vi "FL_Preprocess_and_save_incrementally.vi"(0 "Temporary file output path":path, 1 "Loop iteration":i32, 2 "Mouse face dir. swap":bool, 3 "Loop speed in ms":u16, 4 "Save every N seconds":u32=15, 5 "error in (no error)":errorcluster, 6 "Filter type":u16(ring)=5 items=["None", "Kalman 0.50", "Kalman 0.30", "Kalman 0.12", "Savitzky-Golay 3/5", "Savitzky-Golay 3/11", "Savitzky-Golay 3/31"], 7 "Sensor read input":T3(array[cluster]), 8 "Offset":sgl, 9 "tdms file in":refnum<k34>, 10 "Pixels per mm":dbl, 11 "Data flow controls in":T2, 12 "Diagram at recording bounds":T1, 13 "Sensor board size":string="Small") -> (14 "Eff. save interval":sgl, 15 "Latest sensor output (decoded)":string[][](array[string]), 16 "Fire TTL":bool, 17 "TTL out N":u8, 18 "Current TTL status":u8, 19 "error out":errorcluster)   [LabVIEW 2018, in "Tracker.lvlib"]
uses:
  Tracker.lvlib
  SW_Globals.vi
  <vilib>/Utility/miscctls.llb/LVBoundsTypeDef.ctl
  <vilib>/Utility/file.llb/Write Delimited Spreadsheet (string).vi
panel:
  out "Bytes return count":u32
  out "VISA error out":errorcluster
  out "Output to the external terminal":string
  in  "Max chunk size":i64=100000
  in  "Number of the file chunk":u32
  out "Chunk size (in bytes)":i64
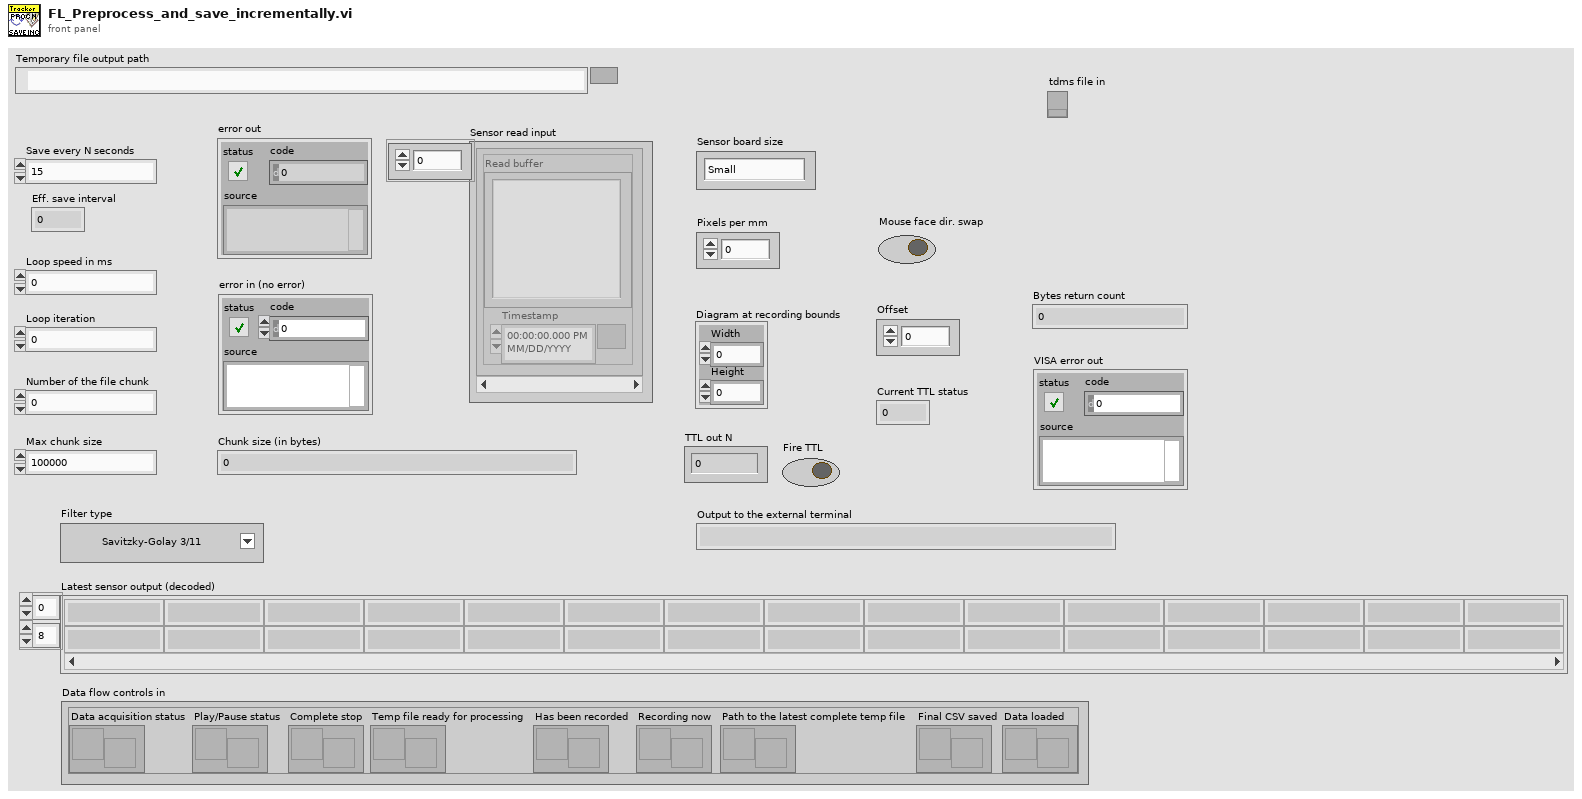
[diagram p1: front panel]
types:
  T1 = typedef "LVBoundsTypeDef.ctl" = cluster{"Width":u32, "Height":u32}
  T2 = cluster{"Data acquisition status":refnum<notifier>, "Play/Pause status":refnum<notifier>, "Complete stop":refnum<notifier>, "Temp file ready for processing":refnum<notifier>, "Has been recorded":refnum<notifier>, "Recording now":refnum<notifier>, "Path to the latest complete temp file":refnum<notifier>, "Final CSV saved":refnum<notifier>, "Data loaded":refnum<notifier>}
  T3 = cluster{"Read buffer":string, "Timestamp":timestamp}[]
  T4 = cluster{"ms since ON":u32, "delta time":u32, "X1":sgl, "Y1":sgl, "X2":sgl, "Y2":sgl, "TTL inputs":u8, "TTL outputs":u8, "Frame timestamp":timestamp, "Frame OK":bool}
  T5 = cluster{"X1 filtered":dbl, "Y1 filtered":dbl, "X2 filtered":dbl, "Y2 filtered":dbl, "X1 raw":dbl, "Y1 raw":dbl, "X2 raw":dbl, "Y2 raw":dbl}
  T6 = cluster{"R from center":dbl, "sin(a)":dbl, "Mouse Xc":dbl, "Mouse Yc":dbl, "X1-X2":dbl, "Y1-Y2":dbl, "Cage Xc":dbl, "Cage Yc":dbl}
  T7 = cluster{"R from center":dbl, "phi (mouse angular position in the cage)":dbl, "alpha (mouse rot. angle)":sgl, "X":dbl, "Y":dbl, "theta (from center towards mouse)":dbl, "beta (cage rot. against mouse)":sgl, "w (mouse angle to wall)":dbl}
  T8 = cluster{"Zone[1]":bool, "Zone[2]":bool, "Zone[3]":bool, "Zone[4]":bool, "Zone[5]":bool, "Zone[6]":bool, "Zone[7]":bool, "Zone[8]":bool, "Zone[9]":bool, "Zone[10]":bool, "Zone[11]":bool, "Zone[12]":bool, "Zone[13]":bool}
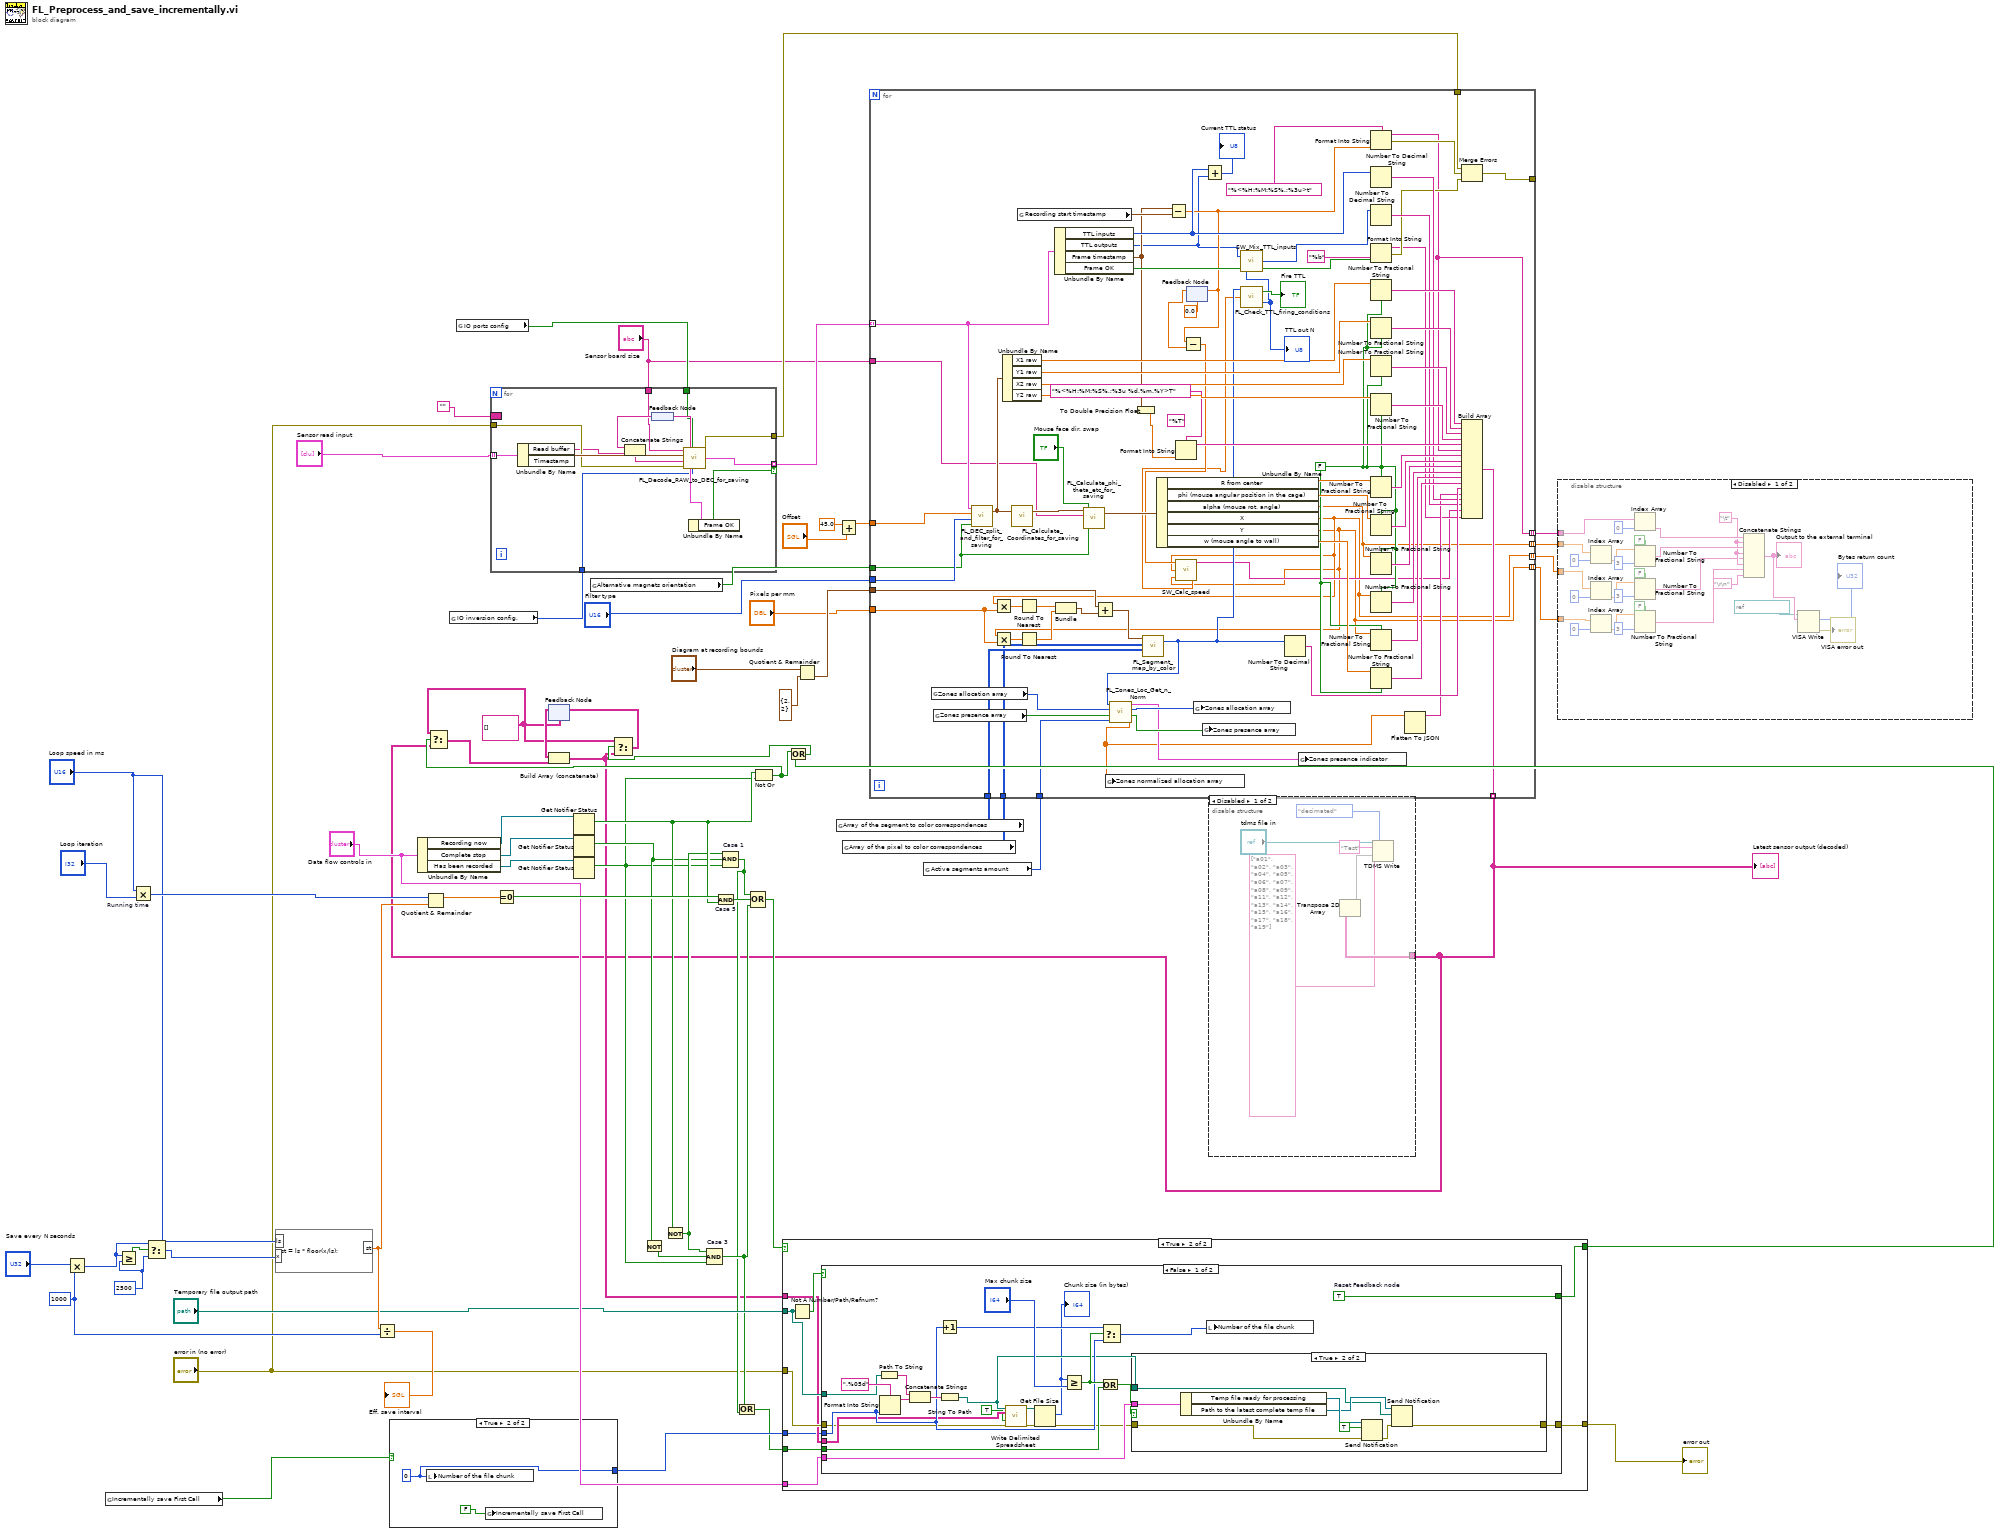
[diagram p0: block diagram]
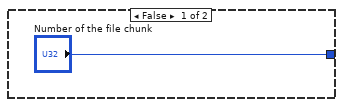
[diagram p4: hidden frame]
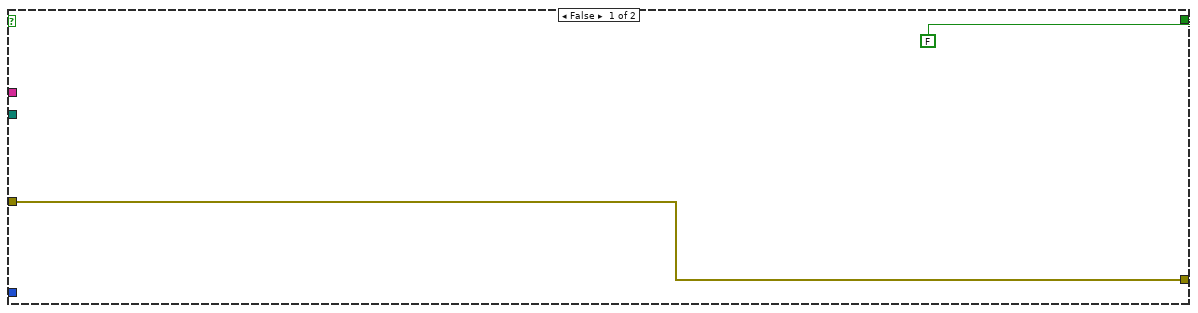
[diagram p5: hidden frame]
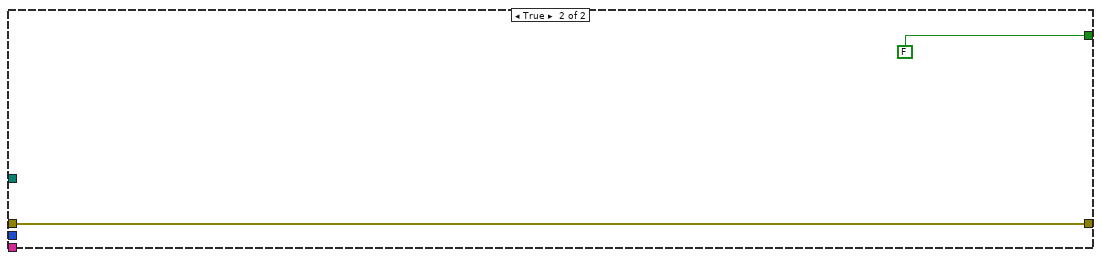
[diagram p7: hidden frame]
diagram:
  w38 = string[][] []
  w51 = u32 1000 ("y")
  w58 = 2500
  n1 = Multiply(x="Save every N seconds", y=w51) -> (x*y=w54:u32)
  n2 = global read "SW_Globals.vi" "Incrementally save First Call"() -> (w8:bool)
  n3 = Greater Or Equal?(x=w54, y=w58) -> (x >= y?=w59:bool)
  n4 = Multiply "Running time"(x="Loop speed in ms", y="Loop iteration") -> (x*y=w62:i32)
  n5 = Select(t=w54, s=w59, f=w58) -> (s? t:f=w56:u32)
  n6 = formula code="st = ls * floor(x/ls);"("ls"="Loop speed in ms", "x"=w56) -> ("st"=w53:dbl)
  n7 = Divide(x=w53, y=w51) -> (x/y=→"Eff. save interval":dbl)
  n8 = case shown="True" w8 {
    tunnel: ["Number of the file chunk" w67] -> w41
    frame False {
    }
    frame True {
      w67 = 0 ("Number of the file chunk")
      n9 = local write "Number of the file chunk"(w67) -> ()
      n10 = global write "SW_Globals.vi" "Incrementally save First Call"(FALSE ("Incrementally save First Call")) -> ()
    }
  }
  n11 = Unbundle By Name("Data flow controls in") -> ("Recording now"=w46:refnum<notifier>, "Complete stop"=w45:refnum<notifier>, "Has been recorded"=w44:refnum<notifier>)
  n12 = Quotient & Remainder(x=w62, y=w53) -> (x-y*floor(x/y)=w60:dbl)  [unwired: 1 out]
  n13 = global read "SW_Globals.vi" "IO inversion config."() -> (w6:u16)
  n14 = global read "SW_Globals.vi" "IO ports config"() -> (w10:bool[])
  n15 = for {
    tunnel: "Sensor read input" -> [w80] mode=indexing
    border: "" -> [_]
    tunnel: [w75] -> w25 mode=indexing if=w74
    tunnel: [w73] -> w26
    tunnel: "error in (no error)" -> [w72]
    tunnel: "Sensor board size" -> [w71]
    tunnel: w10 -> [w70]
    tunnel: w6 -> [w68]
    n16 = Unbundle By Name(w80) -> ("Read buffer"=w69:string, "Timestamp"=w79:timestamp)
    n17 = feedback #1() -> (w76:string)
    n18 = Concatenate Strings(w76, w69) -> (w78:string)
    n19 = call "FL_Decode_RAW_to_DEC_for_saving.vi"("Sensor board size"=w71, "IO ports config"=w70, "Input timestamp"=w79, "Input string"=w78, "IO inversion config."=w68, "Error In"=w72) -> ("Output string leftover"=w77:string, "DEC output cluster"=w75:T4, "Error Out"=w73:errorcluster)
    n20 = feedback-in #1(w77) -> ()
    n21 = Unbundle By Name(w75) -> ("Frame OK"=w74:bool)
  }
  n22 = Equal To 0?(x=w60) -> (x = 0?=w61:bool)
  n23 = feedback #2(w38) -> (w49:string[][])
  n24 = Get Notifier Status(notifier=w46) -> (current notification=w35:bool)  [unwired: 1 in, 4 out]
  n25 = Get Notifier Status(notifier=w45) -> (current notification=w33:bool)  [unwired: 1 in, 4 out]
  n26 = Get Notifier Status(notifier=w44) -> (current notification=w32:bool)  [unwired: 1 in, 4 out]
  n27 = global read "SW_Globals.vi" "Alternative magnets orientation"() -> (w9:bool)
  n28 = Not(x=w33) -> (.not. x?=w31:bool)
  n29 = Not(x=w35) -> (.not. x?=w34:bool)
  n30 = Compound Arithmetic op=AND "Case 3"(w34, w31, w32) -> (w40:bool)
  n31 = And "Case 5"(x=w61, y=w35) -> (x .and. y?=w64:bool)
  n32 = Compound Arithmetic op=AND "Case 1"(w34, w33, w32) -> (w29:bool)
  n33 = Or(x=w40, y=w29) -> (x .or. y?=w30:bool)
  n34 = Compound Arithmetic op=OR(w29, w64, w40) -> (w50:bool)
  n35 = Not Or(1:w32, 2:w35) -> (0:w37:bool)
  n36 = Quotient & Remainder(x="Diagram at recording bounds", y=T1 {"Width"=2, "Height"=2}) -> (floor(x/y)=w19:T1)  [unwired: 1 out]
  n37 = global read "SW_Globals.vi" "Array of the segment to color correspondences"() -> (w17:u32[][])
  n38 = Add(x=sgl 45.0, y="Offset") -> (x+y=w12:sgl)
  n39 = global read "SW_Globals.vi" "Array of the pixel to color correspondences"() -> (w16:u32[][])
  n40 = global read "SW_Globals.vi" "Active segments amount"() -> (w14:u8)
  n41 = for {
    tunnel: w25 -> [w157] mode=indexing
    tunnel: [w131] -> _
    tunnel: w26 -> [w130]
    tunnel: [w85] -> w5 mode=indexing
    tunnel: "Filter type" -> [w129]
    tunnel: w19 -> [w122]
    tunnel: "Pixels per mm" -> [w128]
    tunnel: w17 -> [w120]
    tunnel: w16 -> [w119]
    tunnel: w14 -> [w115]
    tunnel: w12 -> [w106]
    tunnel: w9 -> [w91]
    tunnel: "Sensor board size" -> [w90]
    tunnel: [w84] -> w3 mode=indexing
    tunnel: [w83] -> w2 mode=indexing
    tunnel: [w82] -> w1 mode=indexing
    tunnel: [w81] -> w4 mode=indexing
    w133 = FALSE ("use system decimal point (T)")
    (unwired) "%T" ("format string")
    n42 = global read "SW_Globals.vi" "Zones allocation array"() -> (w116:i32[])
    n43 = global read "SW_Globals.vi" "Zones presence array"() -> (w114:bool[])
    n44 = call "FL_DEC_split_and_filter_for_saving.vi"("Alternative magnets orientation"=w91, "Filter type"=w129, "Offset"=w106, "DEC input cluster"=w157) -> ("Magnets coords"=w159:T5)  [unwired: 1 in]
    n45 = Unbundle By Name(w159) -> ("X1 raw"=w150:dbl, "Y1 raw"=w148:dbl, "X2 raw"=w146:dbl, "Y2 raw"=w143:dbl)
    n46 = call "FL_Calculate_Coordinates_for_saving.vi"("Magnets coords in"=w159) -> ("Output cluster of data"=w158:T6)  [unwired: 2 in]
    n47 = global read "SW_Globals.vi" "Recording start timestamp"() -> (w156:timestamp)
    n48 = Unbundle By Name(w157) -> ("TTL inputs"=w102:u8, "TTL outputs"=w87:u8, "Frame timestamp"=w94:timestamp, "Frame OK"=w154:bool)
    n49 = call "FL_Calculate_phi_theta_etc_for_saving.vi"("Use alternative magnets orientation"=w91, "Mouse face dir. swap"="Mouse face dir. swap", "Sensor board size"=w90, "Input cluster of data"=w158) -> ("Output data cluster"=w151:T7)  [unwired: 1 in]
    n50 = To Double Precision Float(number=w94) -> (double precision float=w93:dbl)
    n51 = Unbundle By Name(w151) -> ("R from center"=w142:dbl, "phi (mouse angular position in the cage)"=w140:dbl, "alpha (mouse rot. angle)"=w84:sgl, "X"=w83:dbl, "Y"=w82:dbl, "w (mouse angle to wall)"=w135:dbl)
    n52 = Multiply(x=w83, y=w128) -> (x*y=w127:dbl)
    n53 = Multiply(x=w82, y=w128) -> (x*y=w126:dbl)
    n54 = Round To Nearest(number=w127) -> (nearest integer value=w125:dbl)
    n55 = Round To Nearest(number=w126) -> (nearest integer value=w124:dbl)
    n56 = Bundle(w125, w124) -> (w123:cluster{dbl, dbl})  [unwired: 1 in]
    n57 = Add(x=w122, y=w123) -> (x+y=w121:cluster{dbl, dbl})
    n58 = call "FL_Segment_map_by_color.vi"("Array of the segment to color correspondences"=w120, "Array of the pixel to color correspondences"=w119, "Mouse abs. coordinates, pix"=w121) -> ("Current segment' number"=w104:u32)  [unwired: 1 in, 1 out]
    n59 = call "FL_Zones_Loc_Get_n_Norm.vi"("Amount of active segments"=w115, "Zones presence array in"=w114, "Zones allocation array in"=w116, "Current segment' number"=w104) -> ("Zones normalized allocation array out"=w107:dbl[], "Zones presence array out"=w112:bool[], "Zones allocation array out"=w113:i32[], "Zones presence indicator cluster out"=w111:T8)  [unwired: 4 in]
    n60 = global write "SW_Globals.vi" "Zones normalized allocation array"(w107) -> ()
    n61 = Subtract(x=w94, y=w156) -> (x-y=w98:dbl)
    n62 = Format Into String(format string="%<%H:%M:%S%,;%3u %d.%m.%Y>T", w93) -> (resulting string=w152:string)  [unwired: 2 in, 1 out]
    n63 = feedback-in #3(w98) -> ()
    n64 = feedback #3(0.0) -> (w99:dbl)
    n65 = Subtract(x=w98, y=w99) -> (x-y=w96:dbl)
    n66 = call "SW_Calc_speed.vi"("Y coord, mm"=w82, "X coord, mm"=w83, "Time per frame, s"=w96) -> ("Mouse speed for TTL detection, mm/s"=w89:dbl, "Mouse speed for saving, mm/s"=w95:string)  [unwired: 1 out]
    n67 = global write "SW_Globals.vi" "Zones allocation array"(w113) -> ()
    n68 = global write "SW_Globals.vi" "Zones presence array"(w112) -> ()
    n69 = Add(x=w102, y=w87) -> (x+y=→"Current TTL status":u8)
    n70 = call "FL_Check_TTL_firing_conditions.vi"("Current speed, mm/s"=w89, "Current segment' number (last value)"=w104) -> ("TTL out N"=w86:u8, "Fire TTL"=→"Fire TTL":bool)  [unwired: 1 in]
    "TTL out N" <- w86
    n71 = call "SW_Mix_TTL_inputs.vi"("TTL input 2"=w86, "TTL input 1"=w87) -> ("TTL mixed output"=w88:u8)
    n72 = Number To Decimal String(number=w104) -> (decimal integer string=w118:string)  [unwired: 1 in]
    n73 = global write "SW_Globals.vi" "Zones presence indicator"(w111) -> ()
    n74 = Format Into String(format string="%<%H:%M:%S%.;%3u>t", w98) -> (resulting string=w81:string, error out=w132:errorcluster)  [unwired: 2 in]
    n75 = Number To Decimal String(number=w102) -> (decimal integer string=w109:string)  [unwired: 1 in]
    n76 = Number To Decimal String(number=w88) -> (decimal integer string=w110:string)  [unwired: 1 in]
    n77 = Format Into String(format string="%b", w154) -> (resulting string=w97:string, error out=w105:errorcluster)  [unwired: 2 in]
    n78 = Number To Fractional String(use system decimal point (T)=w133, number=w150) -> (F-format string=w149:string)  [unwired: 2 in]
    n79 = Number To Fractional String(use system decimal point (T)=w133, number=w148) -> (F-format string=w147:string)  [unwired: 2 in]
    n80 = Number To Fractional String(use system decimal point (T)=w133, number=w146) -> (F-format string=w145:string)  [unwired: 2 in]
    n81 = Number To Fractional String(use system decimal point (T)=w133, number=w143) -> (F-format string=w144:string)  [unwired: 2 in]
    n82 = Number To Fractional String(use system decimal point (T)=w133, number=w142) -> (F-format string=w141:string)  [unwired: 2 in]
    n83 = Number To Fractional String(use system decimal point (T)=w133, number=w140) -> (F-format string=w139:string)  [unwired: 2 in]
    n84 = Number To Fractional String(use system decimal point (T)=w133, number=w84) -> (F-format string=w138:string)  [unwired: 2 in]
    n85 = Number To Fractional String(use system decimal point (T)=w133, number=w83) -> (F-format string=w137:string)  [unwired: 2 in]
    n86 = Number To Fractional String(use system decimal point (T)=w133, number=w82) -> (F-format string=w136:string)  [unwired: 2 in]
    n87 = Number To Fractional String(use system decimal point (T)=w133, number=w135) -> (F-format string=w134:string)  [unwired: 2 in]
    n88 = Flatten To JSON(anything=w107) -> (JSON string=w108:string)  [unwired: 2 in, 1 out]
    n89 = Merge Errors(w130, w132, w105) -> (w131:errorcluster)
    n90 = Build Array(w149, w147, w145, w144, w152, w81, w141, w139, w138, w137, w136, w134, w118, w108, w109, w110, w95, w97) -> (w85:string[])
  }
  "Latest sensor output (decoded)" <- w5
  n91 = Select(t=w38, s=w37, f=w5) -> (s? t:f=w39:string[][])
  n92 = Build Array (concatenate)(w49, w39) -> (w28:string[][])
  n93 = case shown="True" w50 {
    tunnel: "Temporary file output path" -> [_ w169]
    tunnel: [FALSE w168] -> w47
    tunnel: "error in (no error)" -> [w160 w167]
    tunnel: [w160 w166] -> w22
    tunnel: w28 -> [_ w165]
    tunnel: "Data flow controls in" -> [_ w164]
    tunnel: w41 -> [_ w163]
    tunnel: w30 -> [_ w162]
    frame False {
    }
    frame True {
      n94 = Not A Number/Path/Refnum?(number/path/refnum=w169) -> (NaN/Path/Refnum?=w170:bool)
      n95 = case shown="False" w170 {
        tunnel: w169 -> [w185 _]
        tunnel: [w176 FALSE] -> w168
        tunnel: w167 -> [w172 w203]
        tunnel: [w183 w203] -> w166
        tunnel: w165 -> [w178 _]
        tunnel: w163 -> [w180 _]
        tunnel: w164 -> [w190 _]
        tunnel: w162 -> [w181 _]
        frame False {
          w176 = TRUE  # Reset Feedback node
          n96 = Path To String(path=w185) -> (string=w187:string)
          n97 = Format Into String(format string=".%05d", w180) -> (resulting string=w188:string)  [unwired: 2 in, 1 out]
          n98 = Concatenate Strings(w187, w188) -> (w189:string)
          n99 = Increment(x=w180) -> (x+1=w192:u32)
          n100 = String To Path(string=w189) -> (path=w179:path)
          n101 = call-poly <vilib>:"Write Delimited Spreadsheet.vi"("file path (dialog if empty)"=w179, "2D data"=w178, "append to file? (new file:F)"=TRUE, "error in (no error)"=w172) -> ("new file path (Not A Path if cancelled)"=w175:path, "error out"=w174:errorcluster)  [unwired: 10 in]
          n102 = Get File Size(file=w175, error in=w174) -> (size (in bytes)=w171:i64, 0:w173:errorcluster)  [unwired: 1 out]
          "Chunk size (in bytes)" <- w171
          n103 = Greater Or Equal?(x=w171, y="Max chunk size") -> (x >= y?=w184:bool)
          n104 = Or(x=w184, y=w181) -> (x .or. y?=w182:bool)
          n105 = Select(t=w192, s=w184, f=w180) -> (s? t:f=w191:u32)
          n106 = case shown="True" w182 {
            tunnel: w190 -> [_ w202]
            tunnel: w179 -> [_ w196]
            tunnel: w173 -> [w194 w198]
            tunnel: [w194 w197] -> w183
            frame False {
            }
            frame True {
              n107 = Unbundle By Name(w202) -> ("Temp file ready for processing"=w201:refnum<notifier>, "Path to the latest complete temp file"=w200:refnum<notifier>)
              n108 = Send Notification(notification=TRUE, notifier=w201, error in (no error)=w198) -> (error out=w199:errorcluster)  [unwired: 1 out]
              n109 = Send Notification(notification=w196, notifier=w200, error in (no error)=w199) -> (error out=w197:errorcluster)  [unwired: 1 out]
            }
          }
          n110 = local write "Number of the file chunk"(w191) -> ()
        }
        frame True {
        }
      }
    }
  }
  "error out" <- w22
  n111 = Or(x=w37, y=w47) -> (x .or. y?=w36:bool)
  n112 = Select(t=w38, s=w36, f=w28) -> (s? t:f=w48:string[][])
  n113 = feedback-in #2(w48) -> ()
  n114 = disable-structure shown="Disabled" {
    disable-tunnel: w5 -> [w209 _]
    frame Disabled {
      n115 = Transpose 2D Array(2D array=w209) -> (transposed array=w205:string[][])
      n116 = TDMS Write(0:"tdms file in", 1:enum16{"decimated", "interleaved"}."decimated" ("data layout (0:decimated)"), 5:"Test" ("group name in (Untitled)"), 7:string[] ["a01", "a02", "a03", "a04", "a05", "a06", "a07", "a08", "a09", "a11", "a12", "a13", "a14", "a15", "a16", "a17", "a18", "a19"] ("channel name(s) in (Untitled)"), 9:w205) -> ()  [unwired: 1 in, 4 out]
    }
    frame Enabled {
    }
  }
  n117 = disable-structure shown="Disabled" {
    disable-tunnel: w4 -> [w237 _]
    disable-tunnel: w3 -> [w232 _]
    disable-tunnel: w2 -> [w231 _]
    disable-tunnel: w1 -> [w230 _]
    frame Disabled {
      w218 = "\t"
      n118 = Index Array(array=w232, index=0) -> (element=w229:sgl)
      n119 = Index Array(array=w231, index=0) -> (element=w224:dbl)
      n120 = Index Array(array=w230, index=0) -> (element=w221:dbl)
      n121 = Index Array(array=w237, index=0) -> (element=w220:string)
      n122 = Number To Fractional String(use system decimal point (T)=FALSE, number=w229, precision (6)=i16 3) -> (F-format string=w219:string)  [unwired: 1 in]
      n123 = Number To Fractional String(use system decimal point (T)=FALSE, number=w224, precision (6)=i16 3) -> (F-format string=w217:string)  [unwired: 1 in]
      n124 = Number To Fractional String(use system decimal point (T)=FALSE, number=w221, precision (6)=i16 3) -> (F-format string=w216:string)  [unwired: 1 in]
      n125 = Concatenate Strings(w220, w218, w219, w218, w217, w218, w216, "\r\n") -> (w214:string)
      "Output to the external terminal" <- w214
      n126 = VISA Write(VISA resource name=refnum<visa-resource-name> "COMTEST", write buffer=w214) -> (return count=→"Bytes return count":u32, error out=→"VISA error out":errorcluster)  [unwired: 1 in, 1 out]
    }
    frame Enabled {
    }
  }
